vi "Init_KCubeInertial.vi"(10 "SerialNumber in":string="97000019", 11 ".NET Refnum in":refnum<k24>(container)) -> (1 "JogMode":i32(ring)=1 items=["Continuous"=1, "Step"=2], 2 "Device":refnum<k24>, 3 ".NET Refnum out":refnum<k24>)   [LabVIEW 2019]
doc: "init and set low-level parameters of inertial motor"
uses:
  D:/Victor Sun/optical trap control/Kinesis/Thorlabs.MotionControl.Controls.dll
  Kinesis/Thorlabs.MotionControl.Controls.dll
  D:/Victor Sun/optical trap control/Kinesis/Thorlabs.MotionControl.KCube.InertialMotorCLI.dll
  Kinesis/Thorlabs.MotionControl.KCube.InertialMotorCLI.dll
panel:
  out "MaxVoltage":i32
  out "StepAcceleration":i32
  out "StepRate":i32
  out "JogAcceleration":i32
  out "JogRate":i32
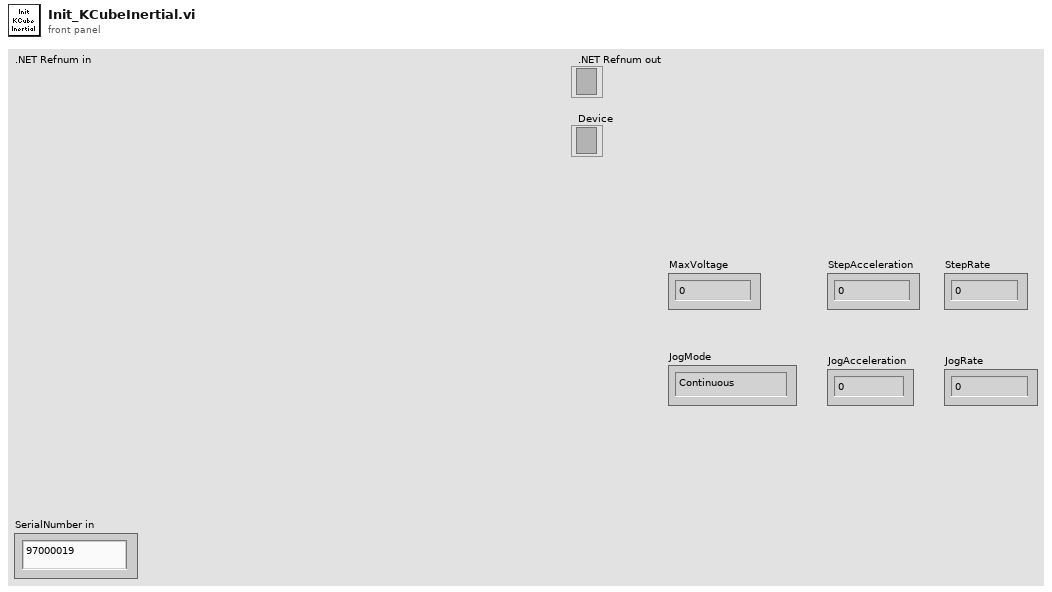
[diagram p1: front panel]
types:
  T1 = cluster{"StepRate":i32, "StepAcceleration":i32, "MaxVoltage":i32}
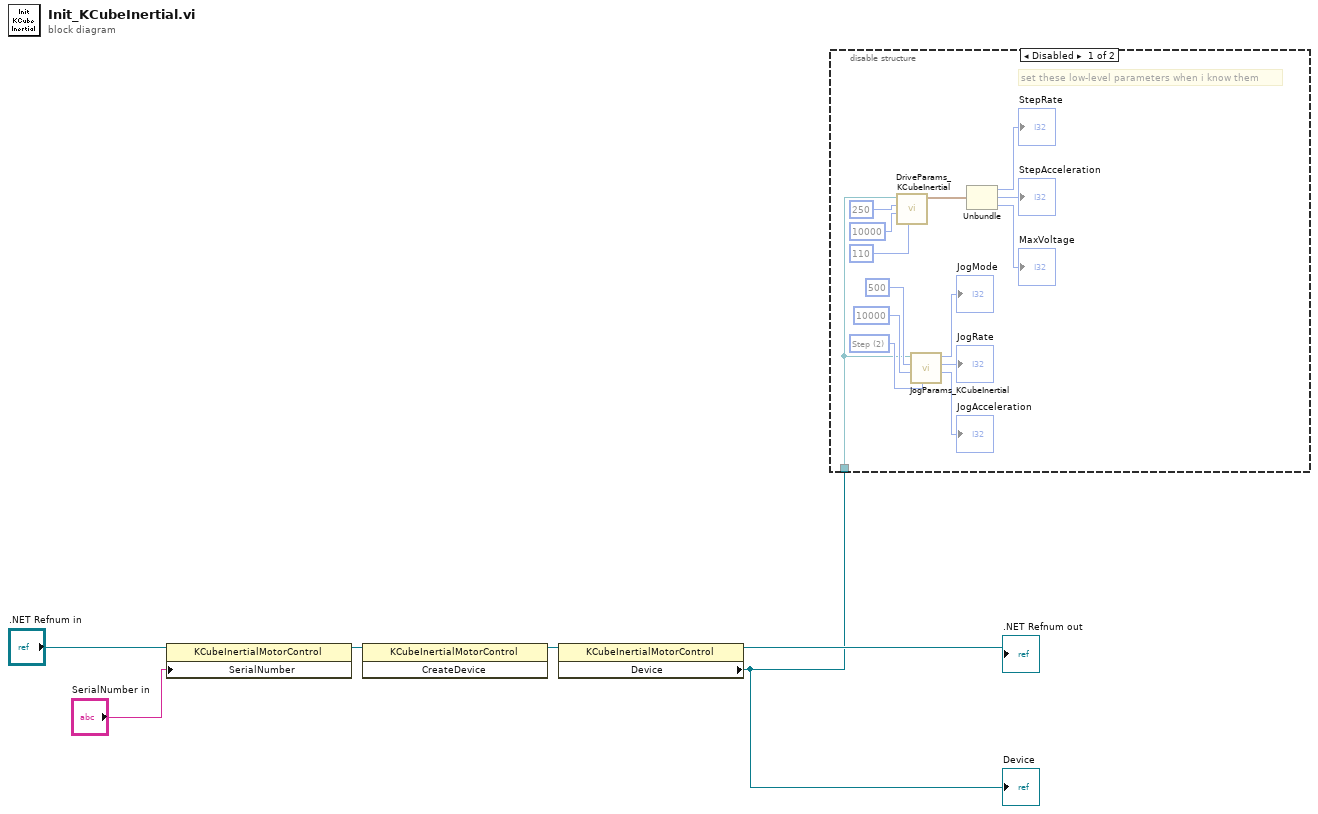
[diagram p0: block diagram]
diagram:
  n1 = property class="KCubeInertialMotorControl"(reference=".NET Refnum in", "SerialNumber"="SerialNumber in") -> (reference out=w3:refnum<k24>)  [unwired: 1 in, 1 out]
  n2 = invoke class="KCubeInertialMotorControl" method="CreateDevice"(reference=w3) -> (reference out=w4:refnum<k24>)  [unwired: 2 in, 2 out]
  n3 = property class="KCubeInertialMotorControl"(reference=w4) -> (reference out=→".NET Refnum out":refnum<k24>, "Device"=w1:refnum<k24>)  [unwired: 1 in, 1 out]
  "Device" <- w1
  n4 = disable-structure shown="Disabled" {
    disable-tunnel: w1 -> [w7 _]
    frame Disabled {
      w10 = 2 items=["Continuous"=1, "Step"=2] ("JogMode")
      # "set these low-level parameters when i know them"
      n5 = call "DriveParams_KCubeInertial.vi"("MaxVoltage"=110, "StepAcceleration"=10000, "StepRate"=250, ".NET Refnum in"=w7) -> ("Cluster"=w17:T1)  [unwired: 7 in]
      n6 = call "JogParams_KCubeInertial.vi"("JogMode in"=w10, "JogAcceleration in"=10000 ("JogAcceleration"), "JogRate in"=500 ("JogRate"), ".NET Refnum in"=w7) -> ("JogAcceleration out"=→"JogAcceleration":i32, "JogRate out"=→"JogRate":i32, "JogMode out"=→"JogMode":i32)  [unwired: 5 in]
      n7 = Unbundle(w17) -> ("StepRate"=→"StepRate":i32, "StepAcceleration"=→"StepAcceleration":i32, "MaxVoltage"=→"MaxVoltage":i32)
    }
    frame Enabled {
    }
  }
